vi "Move Stage.vi"(8 "error in (no error)":errorcluster, 9 "Y Position":dbl, 10 "X Position":dbl, 11 "Recipe Process in":refnum<class "Recipe Process.lvclass">) -> (0 "error out":errorcluster, 3 "Recipe Process out":refnum<class "Recipe Process.lvclass">)   [LabVIEW 2022 SP3, in "Recipe Process.lvlib" / "Recipe Process.lvclass"]
uses:
  Recipe Process.lvclass
  Recipe Process.lvclass/Recipe Process.ctl
  XY Stage/Interfaces/2-Axis Stage API/2-Axis Stage Async API.lvclass
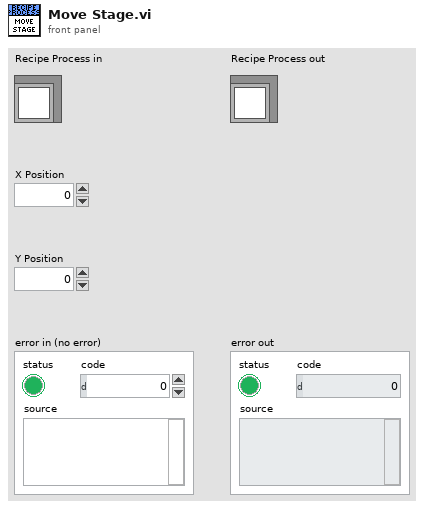
[diagram p1: front panel]
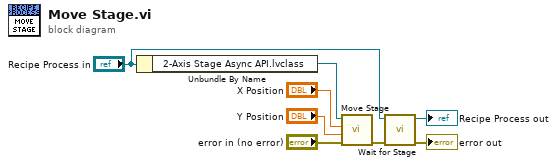
[diagram p0: block diagram]
diagram:
  n1 = Unbundle By Name("Recipe Process in") -> ("2-Axis Stage Async API.lvclass"=w1:refnum<class "2-Axis Stage Async API.lvclass">)
  n2 = call-dynamic "Move Stage.vi"("error in (no error)"="error in (no error)", "Y Axis"="Y Position", "X Axis"="X Position", "2-Axis Stage in"=w1) -> ("error out"=w5:errorcluster)  [unwired: 6 in, 1 out]
  n3 = call "Wait for Stage.vi"("error in (no error)"=w5, "Recipe Process in"="Recipe Process in") -> ("error out"=→"error out":errorcluster, "Recipe Process out"=→"Recipe Process out":refnum<class "Recipe Process.lvclass">)  [unwired: 8 in]
